vi "(SubVI)I2C_16Bit-8Bit_Write_Sequential.vi"(5 "Log Ref":refnum<vi>, 7 "Clock":T1=enum."400kHz", 8 "error in (no error)":errorcluster caption="에러 입력(에러 없음)", 9 "Data to Write":u8[](array[numeric]), 10 "Start Address":u16, 11 "ID":u8) -> (0 "error out":errorcluster caption="에러 출력", 2 "Log":string)   [LabVIEW 2020]
uses:
  Controls/(Ctrl)I2C_Clock.ctl
  Controls/(Ctrl)I2C_RW.ctl
  Controls/(Ctrl)I2C_Data Size.ctl
  Serial/Controls/(Ctrl)Serial_Write Read Option.ctl
  Variables/(Var)System Variables.vi
  Serial/Instance VIs/(SubVI)Serial_Write-Read.vi
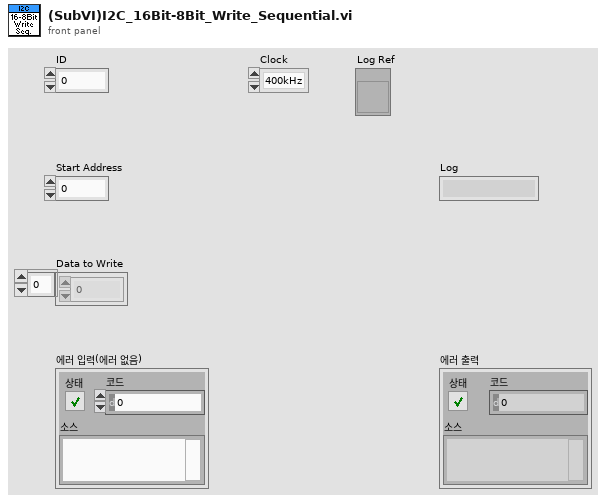
[diagram p1: front panel]
types:
  T1 = typedef "(Ctrl)I2C_Clock.ctl" = enum8{"1MHz", "2MHz", "3MHz", "400kHz"}
  T2 = typedef "(Ctrl)I2C_Data Size.ctl" = enum16{"8Bit_8Bit", "16Bit_16Bit", "16Bit_8Bit"}
  T3 = typedef "(Ctrl)I2C_RW.ctl" = enum16{"Read", "Write"}
  T4 = typedef "(Ctrl)Serial_Write Read Option.ctl" = cluster{"Echo Request":bool, "Header Verification":bool, "Checksum Verification":bool, "User Code Verifiaction":bool}
  T5 = typedef "IC I2C Clock Rate.ctl" = enum8{"50khz", "100khz", "400khz", "1Mhz", "1.2Mhz"}
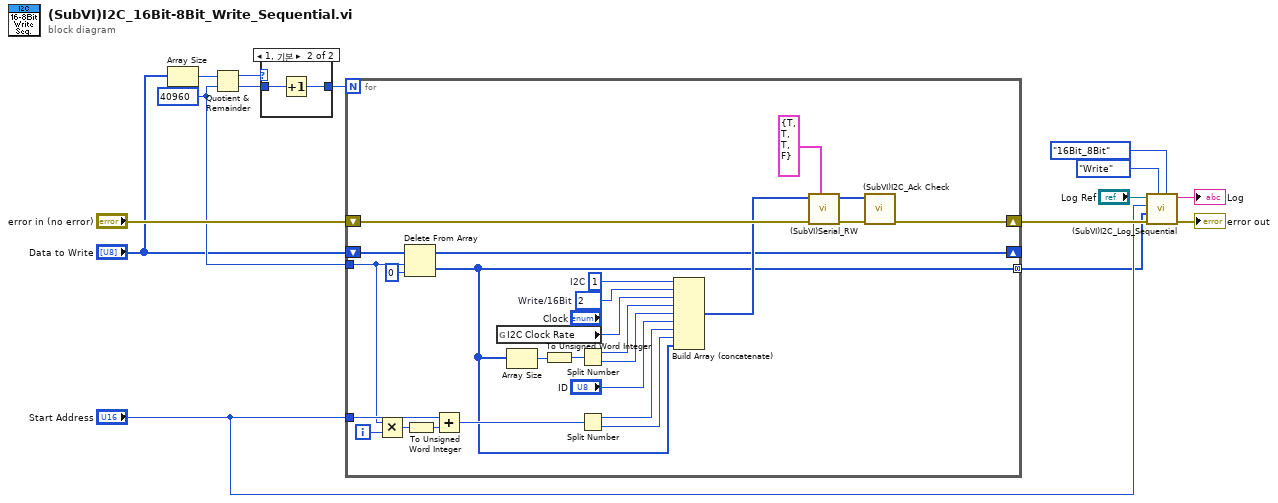
[diagram p0: block diagram]
diagram:
  w3 = 40960 ("y")
  n1 = Array Size(array="Data to Write") -> (size(s)=w7:i32)
  n2 = Quotient & Remainder(x=w7, y=w3) -> (x-y*floor(x/y)=w6:i32, floor(x/y)=w5:i32)
  n3 = case shown="1, 기본" w6 {
    tunnel: w5 -> [w16 w18]
    tunnel: [w16 w17] -> w4
    frame 0 {
    }
    frame 1, Default {
      n4 = Increment(x=w18) -> (x+1=w17:i32)
    }
  }
  n5 = for {
    N: w4 -> [_]
    tunnel: "Start Address" -> [w24]
    shift-right: [w36] -> w14
    shift-left: "error in (no error)" -> [w44]
    tunnel: w3 -> [w21]
    shift-right: [w27] -> _
    shift-left: "Data to Write" -> [w29]
    tunnel: [w20] -> w1 mode=concatenating
    i -> [w26]
    w41 = u8 2  # Write/16Bit
    w42 = u8 1  # I2C
    n6 = Multiply(x=w21, y=w26) -> (x*y=w25:i32)
    n7 = Delete From Array(array=w29, length=w21, index=0 ("인덱스")) -> (deleted portion=w20:u8[], array with subset deleted=w27:u8[])
    n8 = To Unsigned Word Integer(number=w25) -> (unsigned 16bit integer=w23:u16)
    n9 = Add(x=w24, y=w23) -> (x+y=w22:u16)
    n10 = global read "(Var)System Variables.vi" "I2C Clock Rate"() -> (w19:T5)
    n11 = Array Size(array=w20) -> (size(s)=w43:i32)
    n12 = To Unsigned Word Integer(number=w43) -> (unsigned 16bit integer=w37:u16)
    n13 = Split Number(x=w37) -> (hi(x)=w40:u8, lo(x)=w39:u8)
    n14 = Split Number(x=w22) -> (hi(x)=w34:u8, lo(x)=w35:u8)
    n15 = Build Array (concatenate)(w42, w41, w19, w40, w39, "ID", w34, w35, w20) -> (w30:u8[])
    n16 = call-poly "(SubVI)Serial_RW.vi"("Option"=T4 {"Echo Request"=TRUE, "Header Verification"=TRUE, "Checksum Verification"=TRUE, "User Code Verifiaction"=FALSE}, "error in (no error)"=w44, "Data to Write"=w30) -> ("error out"=w33:errorcluster, "Read Data"=w31:u8[])  [unwired: 6 in, 1 out]
    n17 = call "(SubVI)I2C_Ack Check.vi"("에러 입력(에러 없음)"=w33, "Read Data"=w31) -> ("에러 출력"=w36:errorcluster)  [unwired: 8 in, 1 out]
  }
  n18 = call "(SubVI)I2C_Log_Sequential.vi"("Data Size"=(Ctrl)I2C_Data_Size."16Bit_8Bit", "R/W"=(Ctrl)I2C_RW."Write", "error in (no error)"=w14, "Data Array"=w1, "Start Address"="Start Address", "Log Ref"="Log Ref") -> ("error out"=→"error out":errorcluster, "Log"=→"Log":string)  [unwired: 4 in]
